vi "Convert Degrees to Radians.vi"(1 "degrees":dbl format="%.3f") -> (0 "radians":dbl format="%.6f")   [LabVIEW 2015]
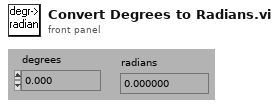
[diagram p1: front panel]
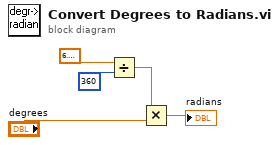
[diagram p0: block diagram]
diagram:
  n1 = Divide(x=6.283185307179586, y=360) -> (x/y=w3:dbl)
  n2 = Multiply(x=w3, y="degrees") -> (x*y=→"radians":dbl)
